vi "Read Key as Array.vi"(7 "section":string, 8 "error in (no error)":errorcluster, 10 "key":string, 11 "refnum":T1) -> (0 "error out":errorcluster, 2 "array":string[](array[string]), 3 "refnum out":T1)   [LabVIEW 2020, in "Utilities.lvlib"]
doc: "Reads a key value of type string from an INI file and converts it to an array of strings. The delimeter is a comma."
uses:
  Utilities.lvlib
  <vilib>/Utility/config.llb/Config Data RefNum.ctl
  <vilib>/Utility/config.llb/Read Key (String).vi
  <vilib>/Utility/config.llb/NI_LVConfig.lvlib
panel:
  in  "read raw string? (F)":bool
  in  "default value":string
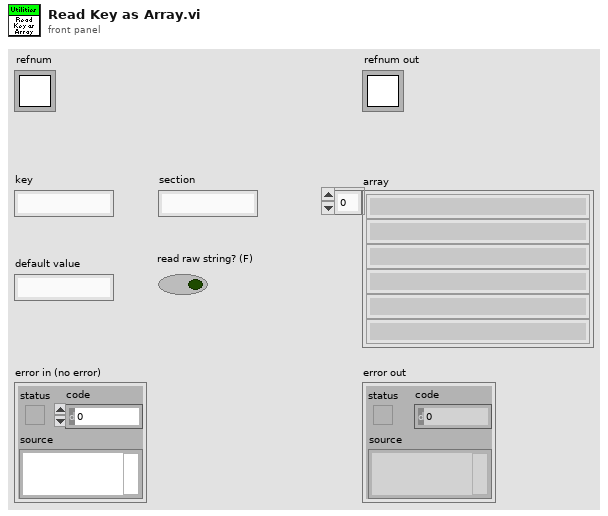
[diagram p1: front panel]
types:
  T1 = typedef "NI_LVConfig.lvlib/Config Data RefNum.ctl" = refnum<k1>
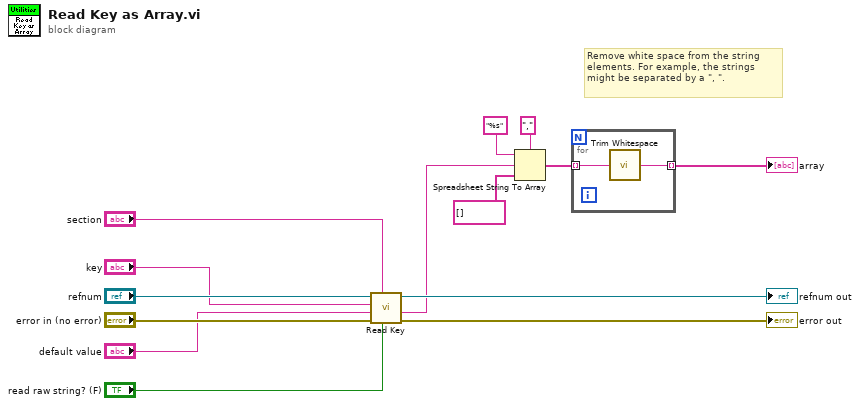
[diagram p0: block diagram]
diagram:
  # "Remove white space from the string elements. For example, the strings might be separated by a \", \"."
  n1 = call-poly <vilib>:"Read Key.vi"("read raw string? (F)"="read raw string? (F)", "section"="section", "error in (no error)"="error in (no error)", "default value"="default value", "key"="key", "refnum"="refnum") -> ("error out"=→"error out":errorcluster, "value"=w6:string, "refnum out"=→"refnum out":T1)  [unwired: 2 in, 1 out]
  n2 = Spreadsheet String To Array(delimiter (Tab)=",", format string="%s", spreadsheet string=w6, array type (2D Dbl)=string[] []) -> (array=w2:string[])
  n3 = for {
    tunnel: w2 -> [w16] mode=indexing
    tunnel: [w15] -> w1 mode=indexing
    n4 = call <vilib>:"Trim Whitespace.vi"("string"=w16) -> ("trimmed string"=w15:string)  [unwired: 1 in]
  }
  "array" <- w1
